vi "GetParent.vi"(8 "error in (no error)":errorcluster, 11 "hWndChild (NULL)":T1) -> (0 "error out":errorcluster, 2 "hWndParent":T1, 3 "dup hWndChild":T1)   [LabVIEW 2011]
doc: "SetParent\nThe SetParent function changes the parent window of the specified child window. \n\nHWND SetParent(\n HWND hWndChild, // handle to window whose parent is changing\n HWND hWndNewParent // handle to new parent window\n);\n \nParameters\nhWndChild \nHandle to the child window. \nhWndNewParent \nHandle to the new parent window. If this parameter is NULL, the desktop window becomes the new parent window. \nWindows NT 5.0 and later: If this parameter is HWND_MESSAGE, the child window becomes a message-only window. \n\nReturn Values\nIf the function succeeds, the return value is a handle to the previous parent window.\n\nIf the function fails, the return value is NULL. To get extended error information, callGetLastError. \n\nRemarks\nAn application can use the SetParent function to set the parent window of a pop-up, overlapped, or child window. The new parent window and the child window must belong to the same application. \n\nIf the window identified by the hWndChild parameter is visible, the system performs the appropriate redrawing and repainting. \n\nFor compatibility reasons, SetParent does not modify the WS_CHILD or WS_POPUP window styles of the window whose parent is being changed. Therefore, if hWndNewParent is NULL, you should also clear the WS_CHILD bit and set the WS_POPUP style after calling SetParent. Conversely, if hWndNewParent is not NULL and the window was previously a child of the desktop, you should clear the WS_POPUP style and set the WS_CHILD style before calling SetParent."
uses:
  hWnd.ctl
  user32.dll
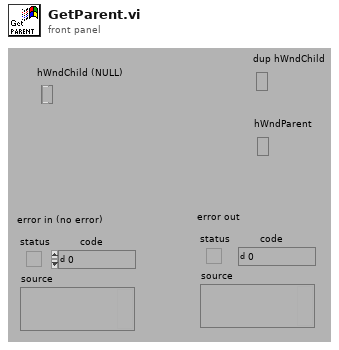
[diagram p1: front panel]
types:
  T1 = typedef "hWnd.ctl" = refnum<k1>
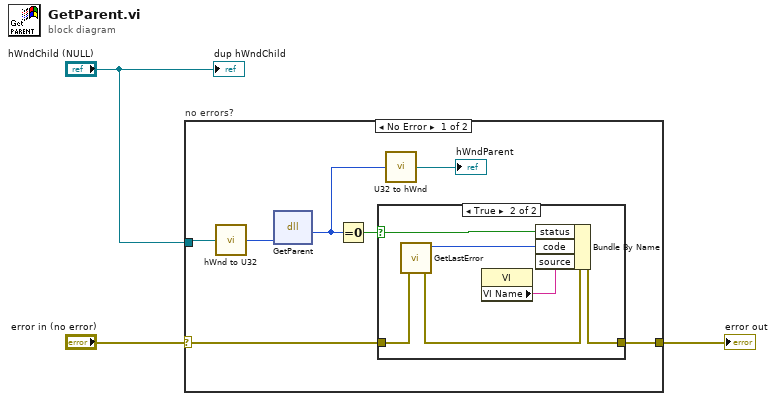
[diagram p0: block diagram]
diagram:
  n1 = case "no errors?" shown="No Error" "error in (no error)" {
    selector: "error in (no error)" -> [w7 w18]
    tunnel: [w8 w18] -> w3
    tunnel: "hWndChild (NULL)" -> [w10 _]
    frame No Error {
      n2 = call "hWnd to U32.vi"("hWnd"=w10) -> ("hWnd"=w9:u32)  [unwired: 4 out]
      n3 = dll-call lib="user32.dll" fn="GetParent"("hWnd"=w9) -> ("hWndParent"=w5:u32)  [unwired: 4 in, 2 out]
      n4 = Equal To 0?(x=w5) -> (x = 0?=w6:bool)
      n5 = case shown="True" w6 {
        selector: w6 -> [_ w12]
        tunnel: w7 -> [w11 w16]
        tunnel: [w11 w17] -> w8
        frame False {
        }
        frame True {
          n6 = call "GetLastError.vi"("error in (no error)"=w16) -> ("error out"=w15:errorcluster, "CODE"=w14:i32)  [unwired: 5 out]
          n7 = property class="VI"() -> ("VI Name"=w13:string)  [unwired: 2 in, 2 out]
          n8 = Bundle By Name(cluster=w15, "status"=w12, "code"=w14, "source"=w13) -> (w17:errorcluster)
        }
      }
      n9 = call "U32 to hWnd.vi"("hWnd"=w5) -> ("hWnd"=→"hWndParent":T1)  [unwired: 4 out]
    }
    frame Error {
    }
  }
  "error out" <- w3
  "dup hWndChild" <- "hWndChild (NULL)"
